vi "文件名读取.vi"(11 "路径":path=path "E:/123") -> (3 "添加的路径":path)   [LabVIEW 2021]
panel:
  in  "文本下拉列表":u16(ring) items=["新建 文本文档 (2)", "新建 文本文档 (3)", "新建 文本文档 (4)", "新建 文本文档"]
  out "数组":string[](array[string])
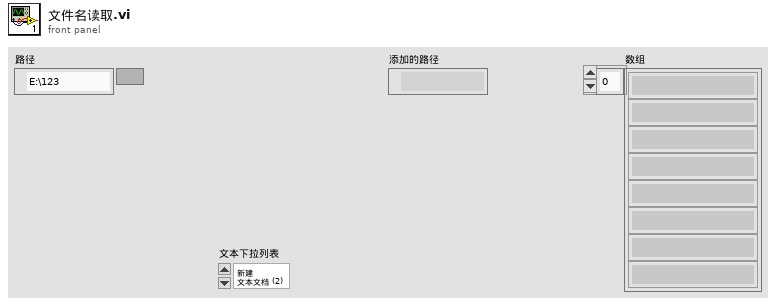
[diagram p1: front panel]
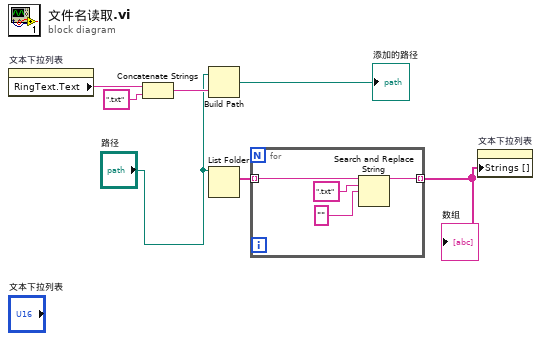
[diagram p0: block diagram]
diagram:
  n1 = property on="文本下拉列表" class="Ring (严格)"() -> ("RingText.Text"=w2:string)  [unwired: 2 in, 2 out]
  n2 = Concatenate Strings(w2, ".txt" ("字符串")) -> (w6:string)
  n3 = Build Path(base path="路径", name or relative path=w6) -> (appended path=→"添加的路径":path)
  n4 = List Folder(path="路径") -> (filenames=w4:string[])  [unwired: 3 in, 3 out]
  n5 = for {
    tunnel: w4 -> [w11] mode=indexing
    tunnel: [w8] -> w3 mode=indexing
    n6 = Search and Replace String(input string=w11, search string=".txt" ("搜索字符串"), replace string="" ("替换字符串(\"\")")) -> (result string=w8:string)  [unwired: 5 in, 3 out]
  }
  "数组" <- w3
  n7 = property on="文本下拉列表" class="Ring (严格)"("Strings []"=w3) -> ()  [unwired: 2 in, 2 out]
